vi "Write Info.vi"(8 "error in (no error)":errorcluster, 10 "Info":T2, 11 "EventsAbstract in":refnum<class "EventsAbstract.lvclass">) -> (0 "error out":errorcluster, 3 "EventsAbstract out":refnum<class "EventsAbstract.lvclass">)   [LabVIEW 2019, in "EventsAbstract.lvclass"]
uses:
  EventsAbstract.lvclass
  SubModules/LogsAbstract/TypeDef/Event Source.ctl
  SubModules/LogsAbstract/LogsAbstract.lvclass
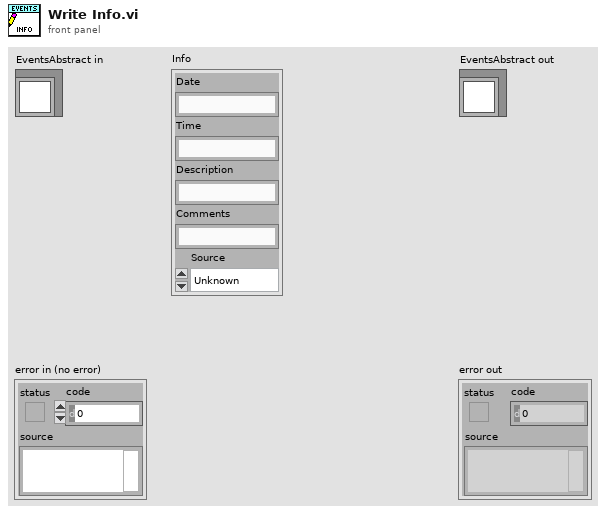
[diagram p1: front panel]
types:
  T1 = typedef "LogsAbstract.lvlib/LogsAbstract.lvclass/Event Source.ctl" = enum16{"Unknown", "< --- Modules --- >", "Core", "< --- SubModules --- >", "Core -> EventLog", "Core -> ErrorLog"}
  T2 = cluster{"Date":string, "Time":string, "Description":string, "Comments":string, "Source":T1}
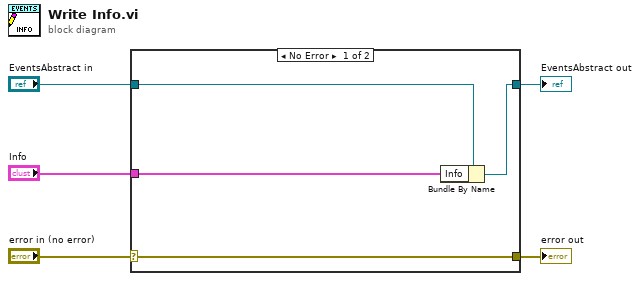
[diagram p0: block diagram]
diagram:
  n1 = case shown="No Error" "error in (no error)" {
    selector: "error in (no error)" -> [w9 w10]
    tunnel: [w9 w10] -> w4
    tunnel: [w7 w11] -> w2
    tunnel: "EventsAbstract in" -> [w8 w11]
    tunnel: "Info" -> [w6 _]
    frame No Error {
      n2 = Bundle By Name(cluster=w8, "Info"=w6) -> (w7:refnum<class "EventsAbstract.lvclass">)
    }
    frame Error {
    }
  }
  "error out" <- w4
  "EventsAbstract out" <- w2
